vi "FCGI parse count.vi"(10 "current index":i32, 11 "unsigned byte array":u8[](array[numeric])) -> (2 "new index":i32, 3 "count":u32)   [LabVIEW 2013]
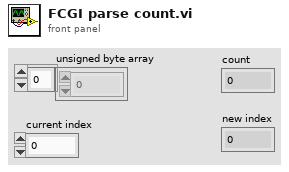
[diagram p1: front panel]
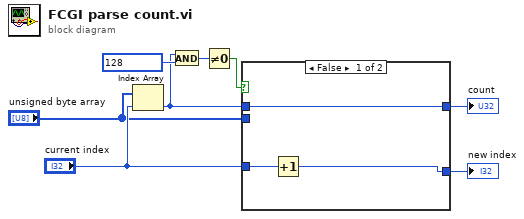
[diagram p0: block diagram]
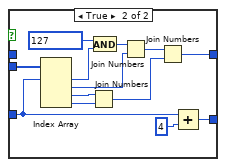
[diagram p2: hidden frame]
diagram:
  n1 = Index Array(array="unsigned byte array", index="current index") -> (element=w5:u8)
  n2 = And(x=w5, y=u8 128) -> (x .and. y?=w1:u8)
  n3 = Not Equal To 0?(x=w1) -> (x != 0?=w2:bool)
  n4 = case shown="False" w2 {
    tunnel: "unsigned byte array" -> [_ w24]
    tunnel: "current index" -> [w11 w16]
    tunnel: w5 -> [w9 _]
    tunnel: [w10 w15] -> w6
    tunnel: [w9 w13] -> w7
    frame False {
      n5 = Increment(x=w11) -> (x+1=w10:i32)
    }
    frame True {
      n6 = Index Array(array=w24, index #1=w16) -> (element #1=w23:u8, element #2=w19:u8, element #3=w18:u8, element #4=w17:u8)  [unwired: 3 in]
      n7 = Join Numbers(hi=w18, lo=w17) -> ((hi.lo)=w21:u16)
      n8 = And(x=u8 127 ("y"), y=w23) -> (x .and. y?=w22:u8)
      n9 = Join Numbers(hi=w22, lo=w19) -> ((hi.lo)=w20:u16)
      n10 = Join Numbers(hi=w20, lo=w21) -> ((hi.lo)=w13:u32)
      n11 = Add(x=w16, y=4) -> (x+y=w15:i32)
    }
  }
  "count" <- w7
  "new index" <- w6
